vi "Pre Analysis Balance.vi"() -> ()   [LabVIEW 2022 SP3]
uses:
  Controls/Setup.ctl
  <vilib>/Analysis/baseanly.llb/A x Vector.vi
  <vilib>/Analysis/baseanly.llb/Mean (DBL).vi
  Globals/Meas_global.vi
  <vilib>/Analysis/NI_AALBase.lvlib
panel:
  out "Raw Data Folders to update":path[](array[path])
  in  "Select Freq Calib file":path
  in  "Calibration File String":string="Joy_13thMay_xls"
  # "Run this vi as a top level to inject setup information into either a Measurement Setup File or Raw Data files."
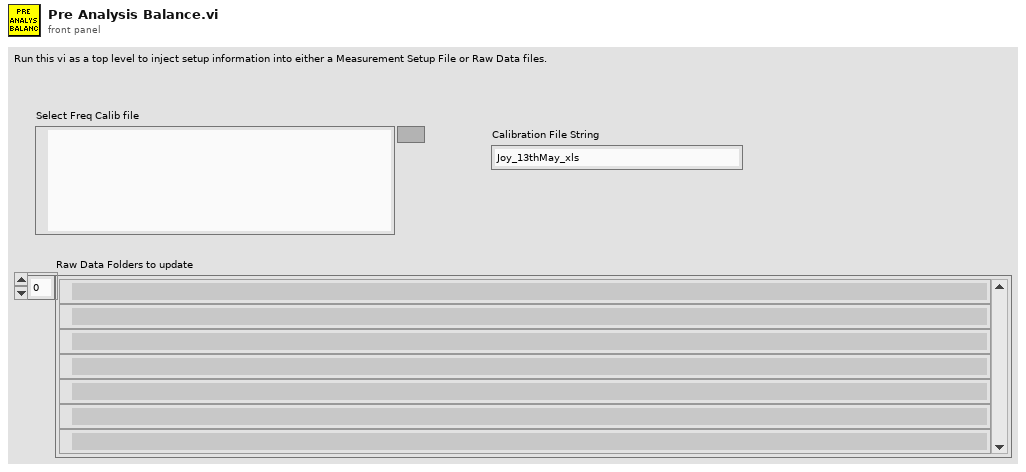
[diagram p1: front panel]
types:
  T1 = typedef "Analysis_info_cluster.ctl" = cluster{"Colour":u32, "Inst type":T2, "Inst name":string, "Symbol":string, "Code name":string, "Extra Info":string, "Inst Array":T3, "Extra Titles":string[], "Extra Values":string[], "U":dbl, "u^2":dbl, "u^3":dbl, "u^4":dbl, "Skew_u":dbl, "Kurt_u":dbl, "Sd Error in Mean":dbl, "% u'/U":dbl, "X":dbl, "Y":dbl, "Z":dbl, "Timescale integral Estimate":dbl, "Sd Error in Variance":dbl, "Calib File":path, "Calib Constants":dbl[], "Output Position":bool, "Stats":enum16{"None", "Basic", "Full"}, "Av Sampling Rate":dbl, "Av No of Samples":dbl, "Total Meas Time (s)":dbl, "ADAM Ch Name":string, "Max value":dbl, "Min value":dbl, "Req Sample Rate Hz":dbl, "Sync Delay Time (s)":dbl, "Ch No":i16, "Device":string, "Use Latest Calib":bool, "Port":string, "Metadata Ch Names":string[], "Metadata Ch Values":string[], "Label":string, "chState":T4}
  T2 = typedef "Inst_type.ctl" = enum16{"Raw voltage", "Raw with zero offsetting", "Propeller anemometer", "Pressure Transducer", "Pitot-static tube", "Hot wire", "Cross wire 1", "Cross wire 2", "Generic Linear", "Generic Polynomial", "Generic BackPoly", "Fast FID", "Thermocouple", "Cold wire", "Pulsed Wire", "LDA Vel", "LDA Tran time", "LDA Arr time", "Microphone"}
  T3 = typedef "Instrument_Array.ctl" = enum16{"PWA", "LDA", "Analogue"}
  T4 = typedef "channelState.ctl" = enum32{"No Selection", "Solo", "Mute"}
  T5 = typedef "Setup.ctl" = enum16{"Run Program", "Show Setup", "Save Current Setup", "Setup Front Panel"}
  T6 = typedef "Time_Trace_Cluster.ctl" = cluster{"Weighting":dbl[], "Voltage":dbl[], "Eng Values":dbl[]}
  T7 = typedef "Post_Process.ctl" = enum16{"Take New Data", "Post Process Raw Data File"}
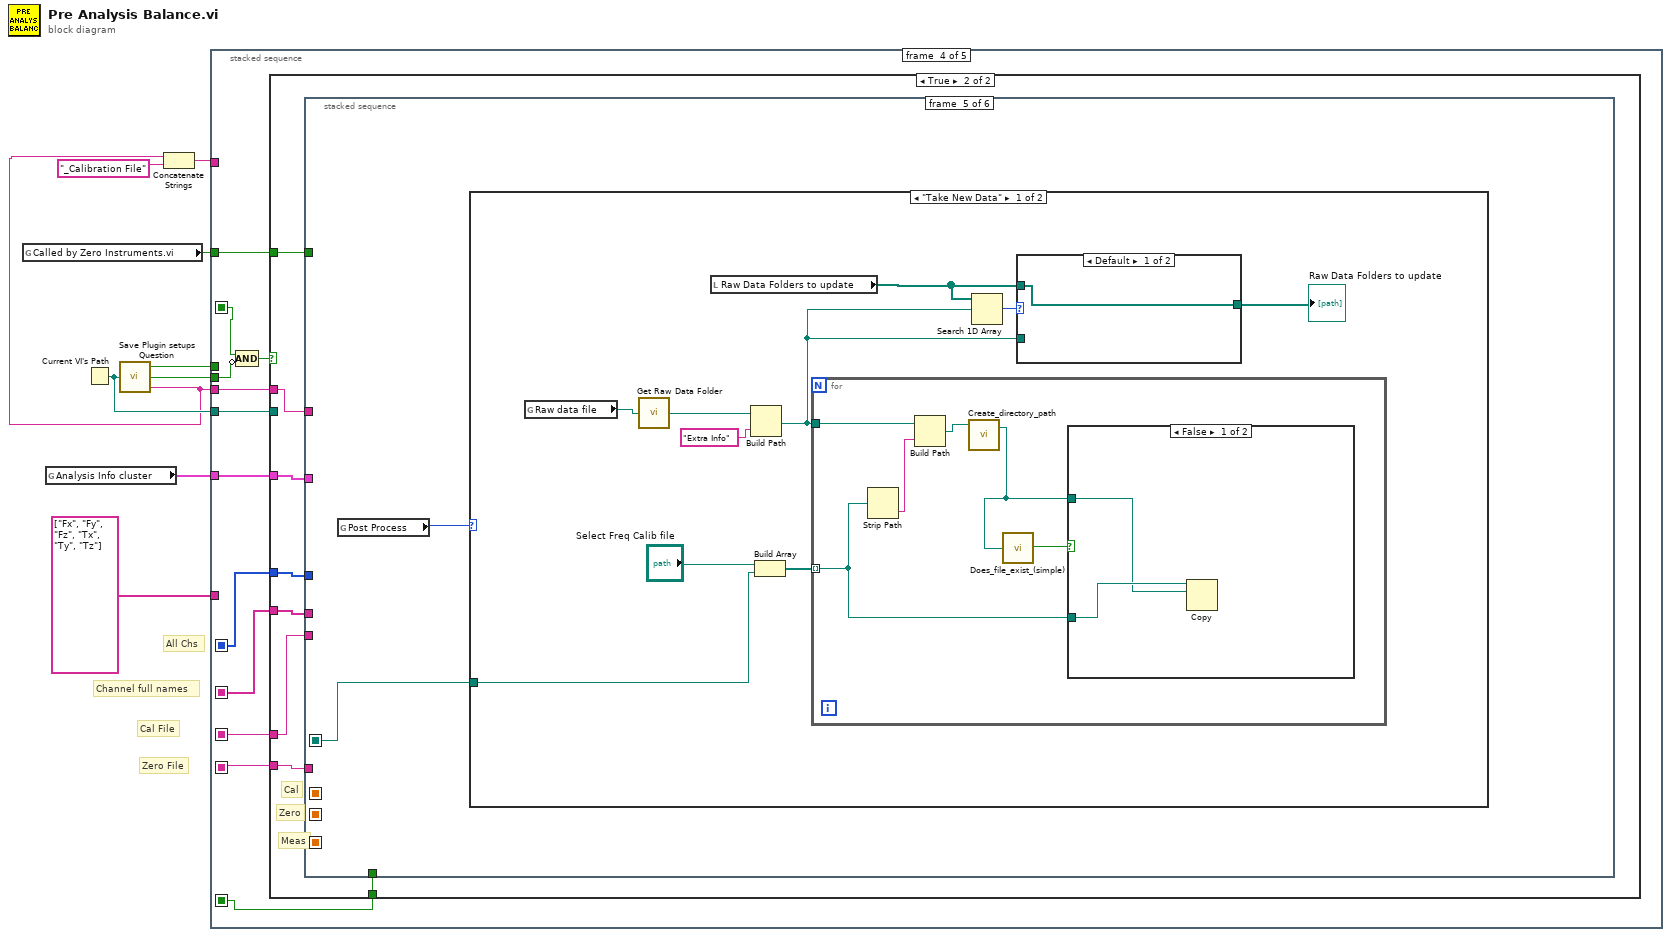
[diagram p0: block diagram]
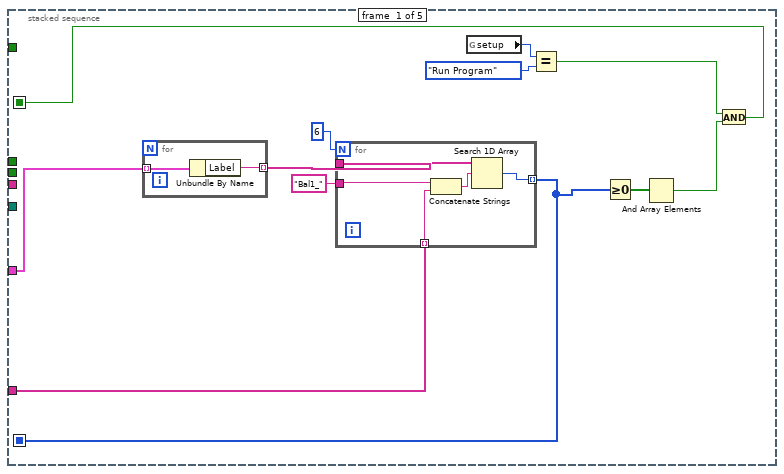
[diagram p2: hidden frame]
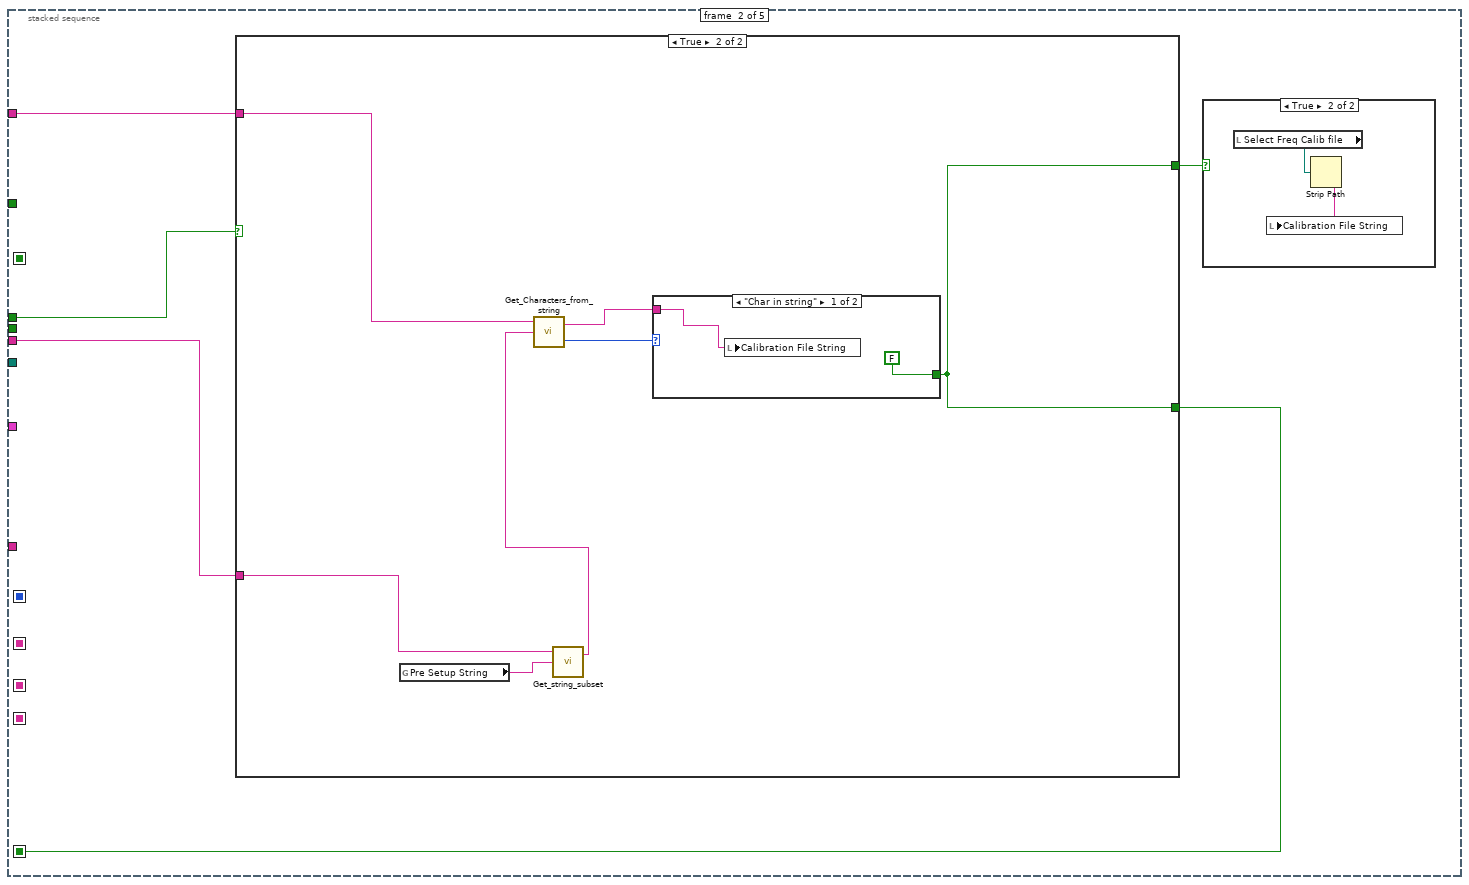
[diagram p3: hidden frame]
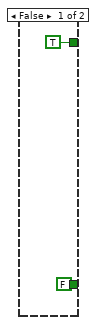
[diagram p5: hidden frame]
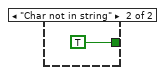
[diagram p6: hidden frame]
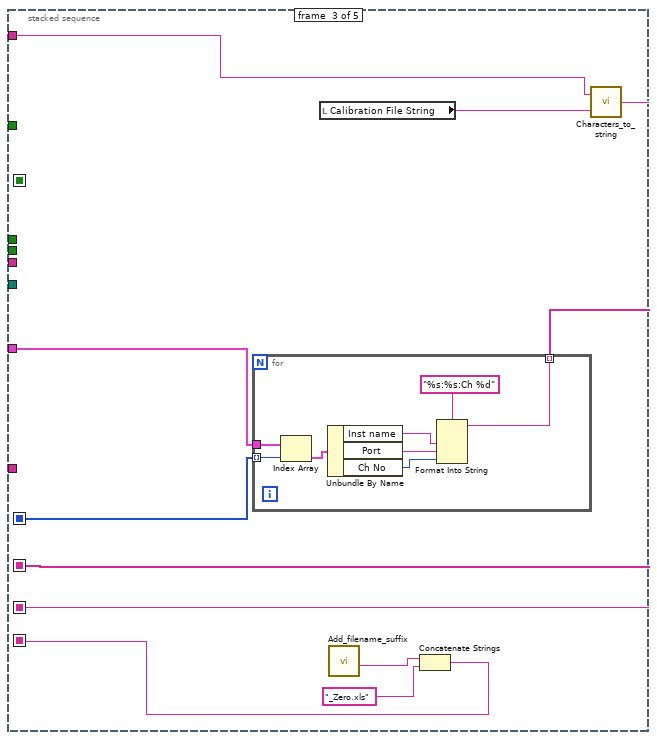
[diagram p7: hidden frame]
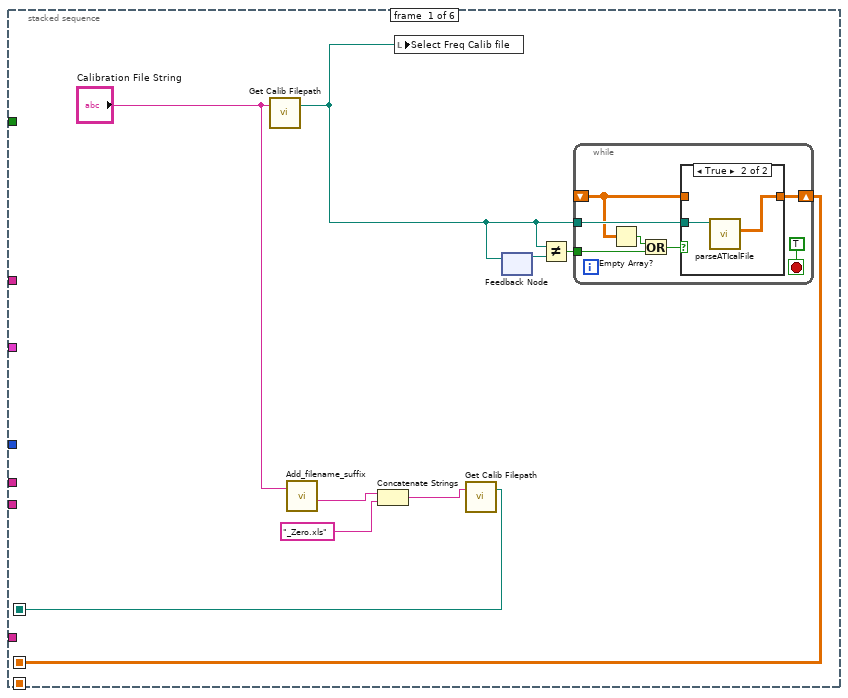
[diagram p9: hidden frame]
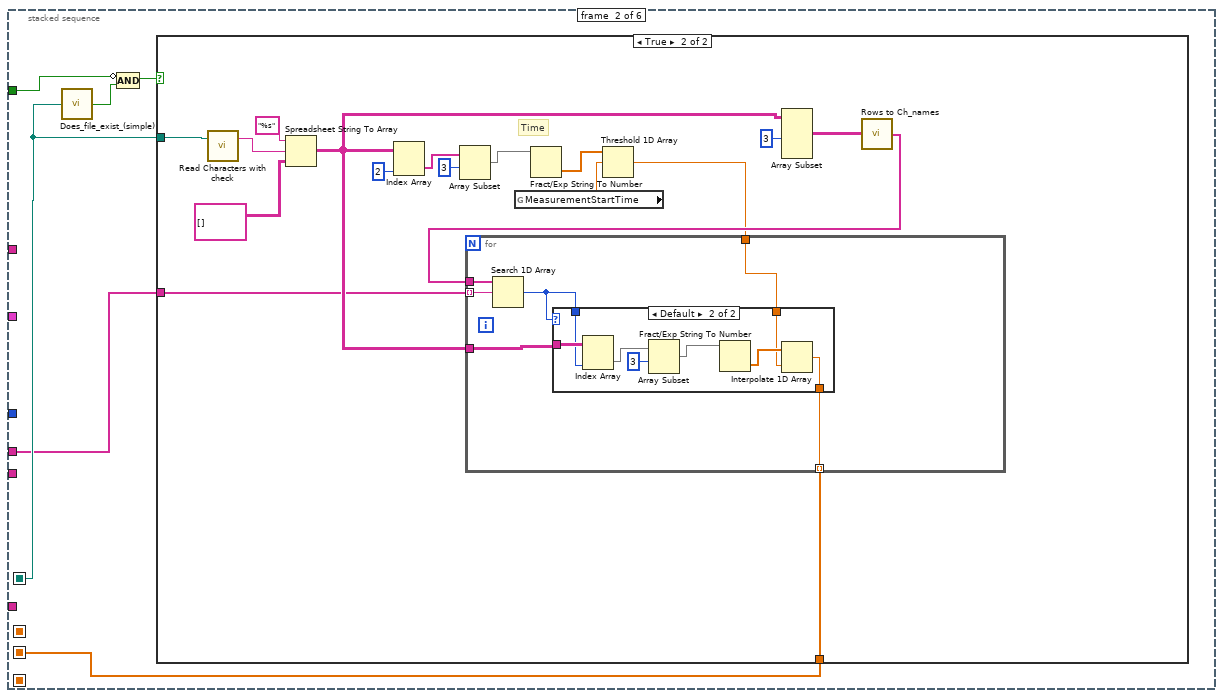
[diagram p11: hidden frame]
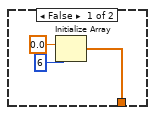
[diagram p12: hidden frame]
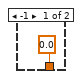
[diagram p13: hidden frame]
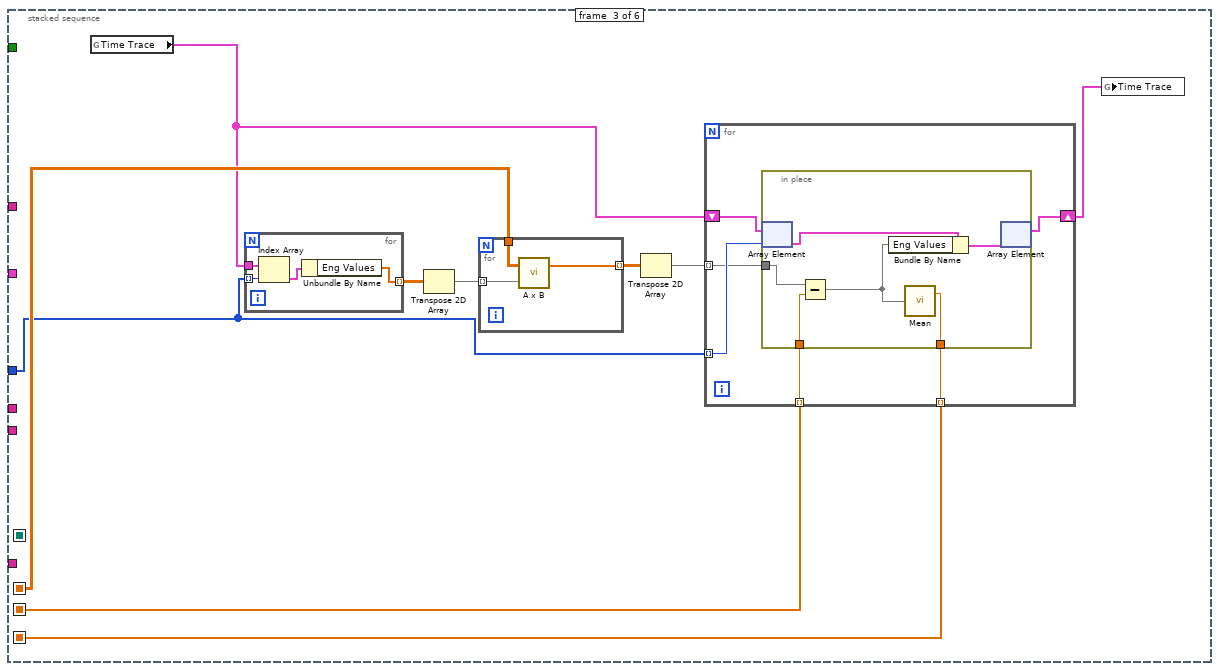
[diagram p14: hidden frame]
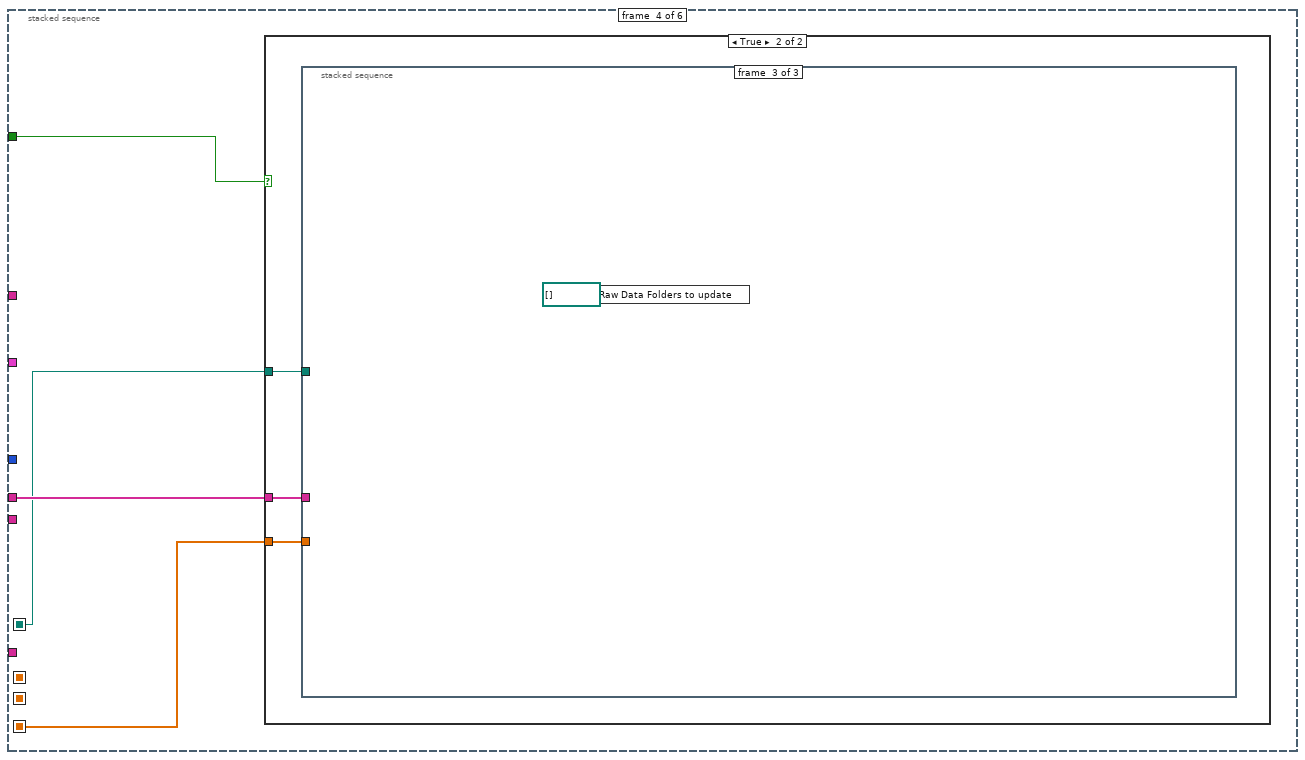
[diagram p15: hidden frame]
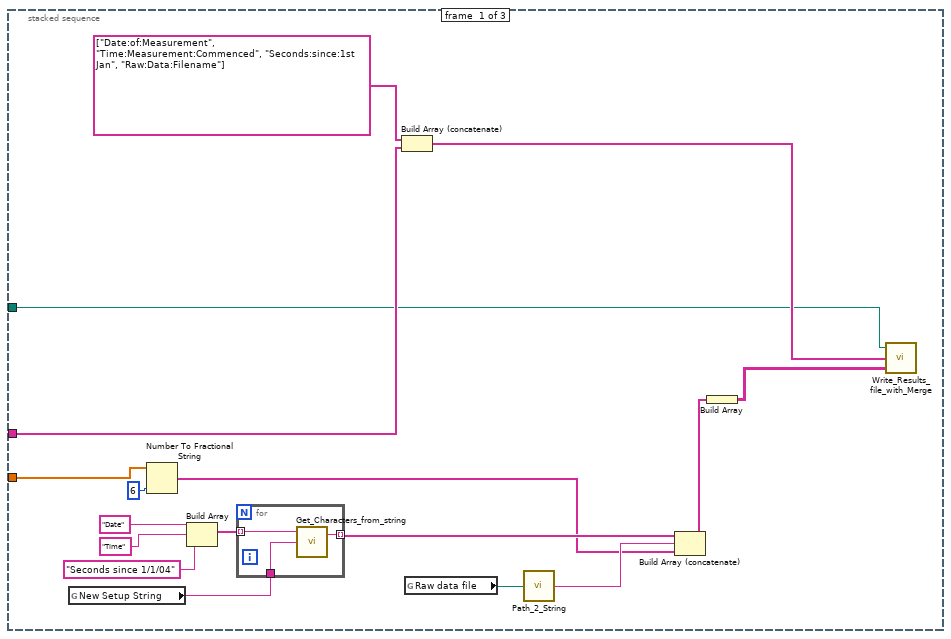
[diagram p17: hidden frame]
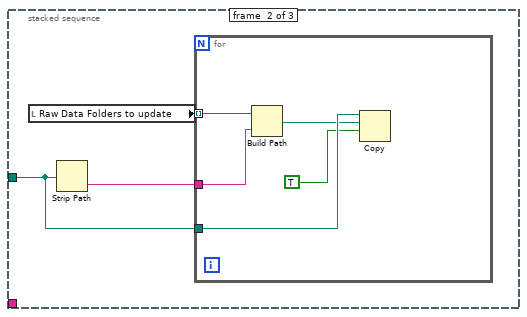
[diagram p18: hidden frame]
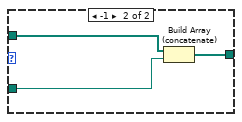
[diagram p19: hidden frame]
diagram:
  # "Channel full names"
  # "Zero File"
  # "Cal File"
  # "All Chs"
  n1 = global read "Meas_global.vi" "Called by Zero Instruments.vi"() -> (w1:bool)
  n2 = global read "Meas_global.vi" "Analysis Info cluster"() -> (w4:T1[])
  n3 = Current VI's Path() -> (path=w5:path)
  n4 = call "Save Plugin setups Question.vi"("VI path"=w5) -> ("Load Plugin Setup"=w9:bool, "Save Plugin Setup"=w6:bool, "Plugin_Label"=w3:string)
  n5 = Concatenate Strings(w3, "_Calibration File" ("string")) -> (w7:string)
  n6 = stacked-sequence {
    seq-local: [w14 _ _ _ _] -> [_ _ w50 w73 _]
    seq-local: [_ _ w52 _ _] -> [_ _ _ w72 w242]
    seq-local: [_ w30 _ _ _] -> [_ _ _ w71 w241]
    seq-local: [w11 _ _ _ _] -> [_ _ _ w68 _]
    seq-local: [_ _ w51 _ _] -> [_ _ _ w67 _]
    seq-local: [_ _ w48 _ _] -> [_ _ _ w66 _]
    tunnel: w9 -> [_ w33 _ _ _]
    tunnel: w3 -> [_ w32 _ w76 w244]
    tunnel: w7 -> [_ w31 w55 _ _]
    tunnel: w6 -> [_ _ _ w70 w245]
    tunnel: w5 -> [_ _ _ w75 w243]
    tunnel: w4 -> [w18 _ w49 w74 _]
    tunnel: string[] ["Fx", "Fy", "Fz", "Tx", "Ty", "Tz"] -> [w10 _ _ _ _]
    tunnel: w1 -> [_ _ _ w65 _]
    frame #0 {
      n7 = for {
        tunnel: w18 -> [w28] mode=indexing
        tunnel: [w27] -> w19 mode=indexing
        n8 = Unbundle By Name(w28) -> ("Label"=w27:string)
      }
      n9 = for {
        N: 6 -> [_]
        tunnel: w19 -> [w26]
        tunnel: "Bal1_" ("element") -> [w25]
        tunnel: [w23] -> w14 mode=indexing
        tunnel: w10 -> [w22] mode=indexing
        n10 = Concatenate Strings(w25, w22) -> (w24:string)
        n11 = Search 1D Array(1D array=w26, element=w24) -> (index of element=w23:i32)  [unwired: 1 in]
      }
      n12 = global read "Meas_global.vi" "setup"() -> (w17:T5)
      n13 = Equal?(x=w17, y=Setup."Run Program" ("setup")) -> (x = y?=w12:bool)
      n14 = Greater Or Equal To 0?(x=w14) -> (x >= 0?=w15:bool[])
      n15 = And Array Elements(Boolean array=w15) -> (logical AND=w13:bool)
      n16 = And(x=w12, y=w13) -> (x .and. y?=w11:bool)
    }
    frame #1 {
      n17 = case shown="True" w33 {
        tunnel: w32 -> [_ w43]
        tunnel: w31 -> [_ w42]
        tunnel: [FALSE w38] -> w30
        tunnel: [TRUE w38] -> w29
        frame False {
        }
        frame True {
          n18 = global read "Meas_global.vi" "Pre Setup String"() -> (w44:string)
          n19 = call "Get_string_subset.vi"("String to split"=w44, "File Label"=w43) -> ("Output string"=w39:string)  [unwired: 2 in, 1 out]
          n20 = call "Get_Characters_from_string.vi"("Input string"=w39, "Variable name"=w42) -> ("Status"=w41:enum16{"Char in string", "Char not in string"}, "Value"=w40:string)  [unwired: 1 in]
          n21 = case shown="\"Char in string\"" w41 {
            tunnel: w40 -> [w46 _]
            tunnel: [FALSE TRUE] -> w38
            frame "Char in string" {
              n22 = local write "Calibration File String"(w46) -> ()
            }
            frame "Char not in string" {
            }
          }
        }
      }
      n23 = case shown="True" w29 {
        frame False {
        }
        frame True {
          n24 = local read "Select Freq Calib file"() -> (w35:path)
          n25 = Strip Path(path=w35) -> (name=w34:string)  [unwired: 1 out]
          n26 = local write "Calibration File String"(w34) -> ()
        }
      }
    }
    frame #2 {
      n27 = for {
        tunnel: w50 -> [w64] mode=indexing
        tunnel: w49 -> [w63]
        tunnel: [w57] -> w48 mode=indexing
        n28 = Index Array(array=w63, index=w64) -> (element=w62:T1)
        n29 = Unbundle By Name(w62) -> ("Inst name"=w58:string, "Port"=w59:string, "Ch No"=w60:i16)
        n30 = Format Into String(format string="%s:%s:Ch %d", w58, w59, w60) -> (resulting string=w57:string)  [unwired: 2 in, 1 out]
      }
      n31 = local read "Calibration File String"() -> (w56:string)
      n32 = call "Add_filename_suffix.vi"() -> ("Base name"=w54:string)  [unwired: 2 in, 3 out]
      n33 = Concatenate Strings(w54, "_Zero.xls" ("Suffix to add")) -> (w51:string)
      n34 = call "Characters_to_string.vi"("Characters to write"=w56, "Label for characters"=w55) -> ("Output string"=w52:string)  [unwired: 1 in]
    }
    frame #3 {
      n35 = Compound Arithmetic op=AND(w68, invert w70) -> (w69:bool)
      n36 = case shown="True" w69 {
        tunnel: w76 -> [_ w82]
        tunnel: w75 -> [_ _]
        tunnel: w74 -> [_ w84]
        tunnel: w73 -> [_ w83]
        tunnel: w72 -> [_ w81]
        tunnel: w71 -> [_ w80]
        tunnel: w67 -> [_ w79]
        tunnel: w66 -> [_ w78]
        tunnel: w65 -> [_ w77]
        frame False {
        }
        frame True {
          # "Meas"
          # "Zero"
          # "Cal"
          n37 = stacked-sequence {
            seq-local: [w90 _ _ _ _ _] -> [_ _ w152 _ _ _]
            seq-local: [_ _ w146 _ _ _] -> [_ _ _ w177 _ _]
            seq-local: [w85 _ _ _ _ _] -> [_ w109 _ w175 w210 _]
            seq-local: [_ w107 _ _ _ _] -> [_ _ w145 _ _ _]
            tunnel: w84 -> [_ _ _ _ _ _]
            tunnel: w83 -> [_ _ w149 _ _ _]
            tunnel: w82 -> [_ _ _ _ _ w236]
            tunnel: w81 -> [_ _ _ _ _ w235]
            tunnel: w80 -> [_ _ _ _ _ w234]
            tunnel: w79 -> [_ _ _ _ _ _]
            tunnel: w78 -> [_ w108 _ w176 _ _]
            tunnel: w77 -> [_ w105 _ w174 _ _]
            frame #0 {
              n38 = call "Get Calib Filepath.vi"("Filename String"="Calibration File String") -> ("Filename Out"=w91:path)  [unwired: 2 in]
              n39 = call "Add_filename_suffix.vi"("Filename"="Calibration File String") -> ("Base name"=w89:string)  [unwired: 1 in, 3 out]
              n40 = Concatenate Strings(w89, "_Zero.xls" ("Suffix to add")) -> (w86:string)
              n41 = local write "Select Freq Calib file"(w91) -> ()
              n42 = call "Get Calib Filepath.vi"("Filename String"=w86) -> ("Filename Out"=w85:path)  [unwired: 2 in]
              n43 = feedback #1() -> (w92:path)  [unwired: 1 in]
              n44 = feedback-in #1(w91) -> ()
              n45 = Not Equal?(x=w91, y=w92) -> (x != y?=w93:bool)
              n46 = while {
                shift-right: [w100] -> w90
                shift-left: _ -> [w96]
                tunnel: w91 -> [w98]
                tunnel: w93 -> [w94]
                stop <- TRUE stop-if-true
                n47 = Empty Array?(array=w96) -> (empty?=w97:bool)
                n48 = Or(x=w97, y=w94) -> (x .or. y?=w95:bool)
                n49 = case shown="True" w95 {
                  tunnel: w98 -> [_ w102]
                  tunnel: [w101 w103] -> w100
                  tunnel: w96 -> [w101 _]
                  frame False {
                  }
                  frame True {
                    n50 = call "parseATIcalFile.vi"("Calibration File"=w102) -> ("Calibration array"=w103:dbl[][])  [unwired: 9 in, 1 out]
                  }
                }
              }
            }
            frame #1 {
              n51 = call "Does_file_exist_(simple).vi"("Pathname"=w109) -> ("exists?"=w106:bool)
              n52 = Compound Arithmetic op=AND(invert w105, w106) -> (w104:bool)
              n53 = case shown="True" w104 {
                tunnel: w109 -> [_ w115]
                tunnel: w108 -> [_ w114]
                tunnel: [w110 w113] -> w107
                frame False {
                  n54 = Initialize Array(0.0 ("element"), 6 ("dimension size")) -> (w110:dbl[])
                }
                frame True {
                  # "Time"
                  n55 = call "Read Characters with check.vi"("file (use dialog)"=w115) -> ("Read String"=w129:string)  [unwired: 1 in, 1 out]
                  n56 = Spreadsheet String To Array(format string="%s", spreadsheet string=w129, array type (2D Dbl)=string[][] []) -> (array=w125:string[][])  [unwired: 1 in]
                  n57 = Index Array(array=w125, index (col)=2 ("disabled index (col)")) -> (element=w120:string[])  [unwired: 1 in]
                  n58 = Array Subset(array=w120, index=3) -> (w118:string[])  [unwired: 1 in]
                  n59 = global read "Meas_global.vi" "MeasurementStartTime"() -> (w123:dbl)
                  n60 = Fract/Exp String To Number(string=w118) -> (number=w122:dbl[])  [unwired: 3 in, 1 out]
                  n61 = Threshold 1D Array(2:w123, 3:w122) -> (0:w124:dbl)  [unwired: 1 in]
                  n62 = Array Subset(array=w125, length (row)=3 ("length")) -> (w127:string[][])  [unwired: 3 in]
                  n63 = call "Rows to Ch_names.vi"("array type (2D Dbl)"=w127) -> ("Array"=w128:string[])
                  n64 = for {
                    tunnel: w125 -> [w135]
                    tunnel: w124 -> [w134]
                    tunnel: w128 -> [w133]
                    tunnel: w114 -> [w132] mode=indexing
                    tunnel: [w130] -> w113 mode=indexing
                    n65 = Search 1D Array(1D array=w133, element=w132) -> (index of element=w131:i32)  [unwired: 1 out]
                    n66 = case shown="Default" w131 {
                      tunnel: w135 -> [_ w141]
                      tunnel: w134 -> [_ w139]
                      tunnel: [0.0 w138] -> w130
                      tunnel: w131 -> [_ w137]
                      frame -1 {
                      }
                      frame Default {
                        n67 = Index Array(array=w141, index (col)=w137) -> (element=w144:string[])  [unwired: 1 in]
                        n68 = Array Subset(array=w144, index=3) -> (w142:string[])  [unwired: 1 in]
                        n69 = Fract/Exp String To Number(string=w142) -> (number=w140:dbl[])  [unwired: 3 in, 1 out]
                        n70 = Interpolate 1D Array(1:w139, 2:w140) -> (0:w138:dbl)
                      }
                    }
                  }
                }
              }
            }
            frame #2 {
              n71 = global read "Meas_global.vi" "Time Trace"() -> (w150:T6[])
              n72 = for {
                tunnel: w149 -> [w173] mode=indexing
                tunnel: w150 -> [w172]
                tunnel: [w170] -> w154 mode=indexing
                n73 = Index Array(array=w172, index=w173) -> (element=w171:T6)
                n74 = Unbundle By Name(w171) -> ("Eng Values"=w170:dbl[])
              }
              n75 = Transpose 2D Array(2D array=w154) -> (transposed array=w153:dbl[][])
              n76 = for {
                tunnel: w152 -> [w169]
                tunnel: w153 -> [w168] mode=indexing
                tunnel: [w167] -> w151 mode=indexing
                n77 = call-poly <vilib>:"A x B.vi"("Vector"=w168, "A"=w169) -> ("A x Vector"=w167:dbl[])  [unwired: 1 out]
              }
              n78 = Transpose 2D Array(2D array=w151) -> (transposed array=w148:dbl[][])
              n79 = for {
                shift-right: [w158] -> w147
                shift-left: w150 -> [w159]
                tunnel: w149 -> [w160] mode=indexing
                tunnel: w148 -> [w157] mode=indexing
                tunnel: [w156] -> w146 mode=indexing
                tunnel: w145 -> [w155] mode=indexing
                n80 = in-place {
                  in-place-border: w157 -> [w163]
                  in-place-border: [w164] -> w156
                  in-place-border: w155 -> [w162]
                  n81 = in-place-array #2(w159, w160) -> (w166:T6)
                  n82 = Subtract(x=w163, y=w162) -> (x-y=w161:dbl[])
                  n83 = Bundle By Name(cluster=w166, "Eng Values"=w161) -> (w165:T6)
                  n84 = call-poly <vilib>:"Mean.vi"("X"=w161) -> ("mean"=w164:dbl)  [unwired: 1 out]
                  n85 = in-place-array #2(w165) -> (w158:T6[])  [unwired: 1 out]
                }
              }
              n86 = global write "Meas_global.vi" "Time Trace"(w147) -> ()
            }
            frame #3 {
              n87 = case shown="True" w174 {
                tunnel: w177 -> [_ w180]
                tunnel: w176 -> [_ w179]
                tunnel: w175 -> [_ w178]
                frame False {
                }
                frame True {
                  n88 = stacked-sequence {
                    tunnel: w180 -> [w187 _ _]
                    tunnel: w179 -> [w182 _ _]
                    tunnel: w178 -> [w181 w203 _]
                    frame #0 {
                      n89 = global read "Meas_global.vi" "New Setup String"() -> (w194:string)
                      n90 = Number To Fractional String(number=w187, precision (6)=i16 6) -> (F-format string=w186:string[])  [unwired: 2 out]
                      n91 = Build Array("Date", "Time", "Seconds since 1/1/04") -> (w193:string[])
                      n92 = for {
                        tunnel: w193 -> [w200] mode=indexing
                        tunnel: w194 -> [w199]
                        tunnel: [w198] -> w190 mode=indexing
                        n93 = call "Get_Characters_from_string.vi"("Input string"=w199, "Variable name"=w200) -> ("Value"=w198:string)  [unwired: 1 in, 1 out]
                      }
                      n94 = Build Array (concatenate)(string[] ["Date:of:Measurement", "Time:Measurement:Commenced", "Seconds:since:1st Jan", "Raw:Data:Filename"] ("Channel names"), w182) -> (w184:string[])
                      n95 = global read "Meas_global.vi" "Raw data file"() -> (w191:path)
                      n96 = call "Path_2_String.vi"("Real Path"=w191) -> ("Path String"=w189:string)
                      n97 = Build Array (concatenate)(w190, w189, w186) -> (w183:string[])
                      n98 = Build Array(w183) -> (w185:string[][])
                      n99 = call "Write_Results_file_with_Merge.vi"("Values In"=w185, "Channel Names in"=w184, "Filename"=w181) -> ()  [unwired: 1 in, 2 out]
                    }
                    frame #1 {
                      n100 = local read "Raw Data Folders to update"() -> (w202:path[])
                      n101 = Strip Path(path=w203) -> (name=w201:string)  [unwired: 1 out]
                      n102 = for {
                        tunnel: w203 -> [w208]
                        tunnel: w202 -> [w207] mode=indexing
                        tunnel: w201 -> [w206]
                        n103 = Build Path(base path=w207, name or relative path=w206) -> (appended path=w205:path)
                        n104 = Copy(9:TRUE ("overwrite (F)"), 10:w205, 11:w208) -> ()  [unwired: 2 in, 3 out]
                      }
                    }
                    frame #2 {
                      n105 = local write "Raw Data Folders to update"(path[] [] ("Raw Data Folders")) -> ()
                    }
                  }
                }
              }
            }
            frame #4 {
              n106 = global read "Meas_global.vi" "Post Process"() -> (w211:T7)
              n107 = case shown="\"Take New Data\"" w211 {
                tunnel: w210 -> [w221 _]
                frame "Take New Data" {
                  n108 = global read "Meas_global.vi" "Raw data file"() -> (w219:path)
                  n109 = call "Get Raw Data Folder.vi"("Raw data file"=w219) -> ("Main Raw Data Folder"=w218:path)
                  n110 = local read "Raw Data Folders to update"() -> (w212:path[])
                  n111 = Build Path(base path=w218, name or relative path="Extra Info") -> (appended path=w214:path)
                  n112 = Build Array("Select Freq Calib file", w221) -> (w216:path[])
                  n113 = for {
                    tunnel: w214 -> [w231]
                    tunnel: w216 -> [w226] mode=indexing
                    n114 = Strip Path(path=w226) -> (name=w230:string)  [unwired: 1 out]
                    n115 = Build Path(base path=w231, name or relative path=w230) -> (appended path=w228:path)
                    n116 = call "Create_directory_path.vi"("Path name"=w228) -> ("Path name Out"=w227:path)  [unwired: 2 in, 1 out]
                    n117 = call "Does_file_exist_(simple).vi"("Pathname"=w227) -> ("exists?"=w229:bool)
                    n118 = case shown="False" w229 {
                      tunnel: w226 -> [w233 _]
                      tunnel: w227 -> [w232 _]
                      frame False {
                        n119 = Copy(10:w232, 11:w233) -> ()  [unwired: 3 in, 3 out]
                      }
                      frame True {
                      }
                    }
                  }
                  n120 = Search 1D Array(1D array=w212, element=w214) -> (index of element=w215:i32)  [unwired: 1 in]
                  n121 = case shown="Default" w215 {
                    tunnel: w214 -> [_ w225]
                    tunnel: [w222 w224] -> w213
                    tunnel: w212 -> [w222 w223]
                    frame Default {
                    }
                    frame -1 {
                      n122 = Build Array (concatenate)(w223, w225) -> (w224:path[])
                    }
                  }
                  "Raw Data Folders to update" <- w213
                }
                frame "Post Process Raw Data File" {
                }
              }
            }
            frame #5 {
              n123 = case shown="True" w234 {
                tunnel: w236 -> [_ w240]
                tunnel: w235 -> [_ w237]
                frame False {
                }
                frame True {
                  n124 = global read "Meas_global.vi" "New Setup String"() -> (w238:string)
                  n125 = call "Replace_data_in_Label_str.vi"("New data string"=w237, "Input string"=w238, "Variable name"=w240) -> ("Appended string"=w239:string)
                  n126 = global write "Meas_global.vi" "New Setup String"(w239) -> ()
                }
              }
            }
          }
        }
      }
    }
    frame #4 {
      n127 = case shown="True" w245 {
        tunnel: w244 -> [_ w253]
        tunnel: w243 -> [_ w252]
        tunnel: w242 -> [_ w251]
        tunnel: w241 -> [_ _]
        frame False {
          # "All"
          # "Hz"
        }
        frame True {
          n128 = local read "Select Freq Calib file"() -> (w247:path)
          n129 = call "Save Plugin Setup String.vi"("Plug In Pathname"=w252, "Setup String to Save"=w251, "PlugIn Label"=w253) -> ("Meas Setup File"=w246:bool, "Raw Data File Written to"=w250:path[])
          n130 = Strip Path(path=w247) -> (name=w249:string)  [unwired: 1 out]
          n131 = for {
            tunnel: w250 -> [w261] mode=indexing
            tunnel: w249 -> [w260]
            shift-right: [w256] -> _
            shift-left: path[] [] -> [w258]
            tunnel: w247 -> [w254]
            tunnel: w246 -> [w255]
            n132 = case shown="True" w255 {
              tunnel: w261 -> [w264 _]
              tunnel: w260 -> [w263 _]
              tunnel: [w262 w269] -> w257
              tunnel: w254 -> [_ w270]
              frame False {
                n133 = call "Get Raw Data Folder.vi"("Raw data file"=w264) -> ("Main Raw Data Folder"=w266:path)
                n134 = Build Path(base path=w266, name or relative path="Extra Info") -> (appended path=w267:path)
                n135 = Build Path(base path=w267, name or relative path=w263) -> (appended path=w265:path)
                n136 = call "Create_directory_path.vi"("Path name"=w265) -> ("Path name Out"=w262:path)  [unwired: 2 in, 1 out]
              }
              frame True {
                n137 = call "Current_Filepath.vi"("Short_Name"="Cal" ("Data Type"), "Filename in"=w270, "Data Type"="Calibrations") -> ("Filename Out"=w269:path)  [unwired: 1 in, 1 out]
              }
            }
            n138 = Search 1D Array(1D array=w258, element=w257) -> (index of element=w259:i32)  [unwired: 1 in]
            n139 = case shown="-1" w259 {
              tunnel: w258 -> [w273 w278]
              tunnel: w257 -> [_ w275]
              tunnel: [w273 w277] -> w256
              tunnel: w254 -> [_ w274]
              frame 0, Default {
              }
              frame -1 {
                n140 = Build Array (concatenate)(w278, w275) -> (w277:path[])
                n141 = call "Does_file_exist_(simple).vi"("Pathname"=w275) -> ("exists?"=w276:bool)
                n142 = case shown="False" w276 {
                  tunnel: w275 -> [w280 _]
                  tunnel: w274 -> [w279 _]
                  frame False {
                    n143 = Copy(10:w280, 11:w279) -> ()  [unwired: 3 in, 3 out]
                  }
                  frame True {
                  }
                }
              }
            }
          }
        }
      }
    }
  }
